vi "Create.vi"(7 "mode settings":variant, 8 "error in":errorcluster, 9 "number of default channels":i32, 10 "channel settings":variant, 11 "thermocouple mode in":refnum<class "Thermocouple Mode.lvclass">) -> (0 "error out":errorcluster, 1 "channels":refnum<class "Channel.lvclass">[](array[class]), 3 "thermocouple mode out":refnum<class "Thermocouple Mode.lvclass">)   [LabVIEW 2020, in "Scan Engine Scripting.lvlib" / "Thermocouple Mode.lvclass"]
uses:
  Thermocouple Mode.lvclass
  Channel Classes/Channel/Channel.lvclass
  Controls/thermocouple channel settings.ctl
  Channel Classes/Thermocouple Channel/Thermocouple Type.ctl
  Channel Classes/Thermocouple Channel/Measurement Units.ctl
  8454f170-3f7b-42b7-aa7d-eb22b487b2d0.vi
  Channel Classes/Thermocouple Channel/Thermocouple Channel.lvclass
  C:/jenkins/workspace/ercat-custom-device_release_20.4/Custom Device Source/Scripting/Modules/Channel Classes/Channel/Channel.lvclass
  Scan Engine Scripting.lvlib
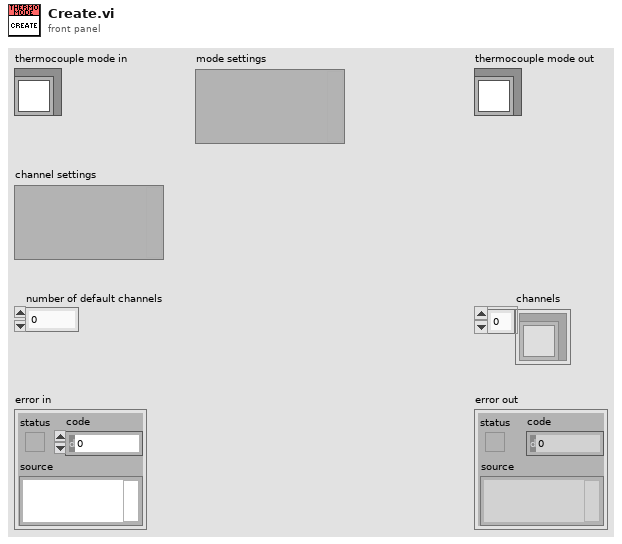
[diagram p1: front panel]
types:
  T1 = typedef "Scan Engine Scripting.lvlib/thermocouple channel settings.ctl" = cluster{"name":string, "default value":dbl, "thermocouple type":T2, "measurement units":T3}
  T2 = typedef "Scan Engine Scripting.lvlib/Thermocouple Channel.lvclass/Thermocouple Type.ctl" = enum16{"J", "K", "T", "E", "R", "S", "N", "B"}
  T3 = typedef "Scan Engine Scripting.lvlib/Thermocouple Channel.lvclass/Measurement Units.ctl" = enum16{"Raw Volts", "Degrees Kelvin", "Degrees Celsius", "Degrees Fahrenheit", "Degrees Rankine"}
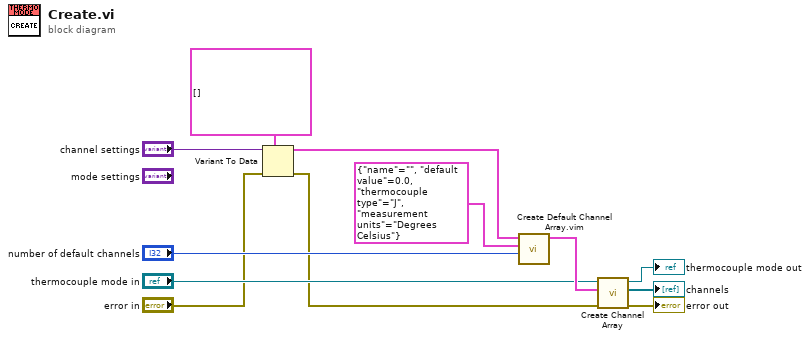
[diagram p0: block diagram]
diagram:
  n1 = Variant To Data(error in="error in", type=T1[] [] ("channel settings in"), Variant="channel settings") -> (data=w6:T1[], error out=w1:errorcluster)
  n2 = call "Create Default Channel Array.vim"("number of default channels"="number of default channels", "default settings"=T1 {"name"="", "default value"=0.0, "thermocouple type"=enum."J", "measurement units"=enum."Degrees Celsius"} ("channel settings"), "channel settings in"=w6) -> ("channel settings out"=w8:T1[])  [unwired: 8 in]
  n3 = call "Create Channel Array.vi"("error in"=w1, "channel settings"=w8, "thermocouple mode in"="thermocouple mode in") -> ("error out"=→"error out":errorcluster, "channels"=→"channels":refnum<class "Thermocouple Channel.lvclass">[], "thermocouple mode out"=→"thermocouple mode out":refnum<class "Thermocouple Mode.lvclass">)  [unwired: 6 in]
